vi "XYZStage-move command constructor.vi"(6 "Bypass Z-safety interlock":bool, 9 "Z":sgl, 10 "Y":sgl, 11 "X":sgl) -> (0 "Move command":string, 1 "Adjusted Z":sgl, 2 "Adjusted Y":sgl, 3 "Adjusted X":sgl)   [LabVIEW 2013]
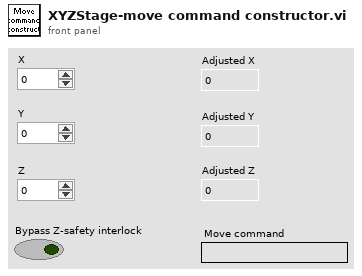
[diagram p1: front panel]
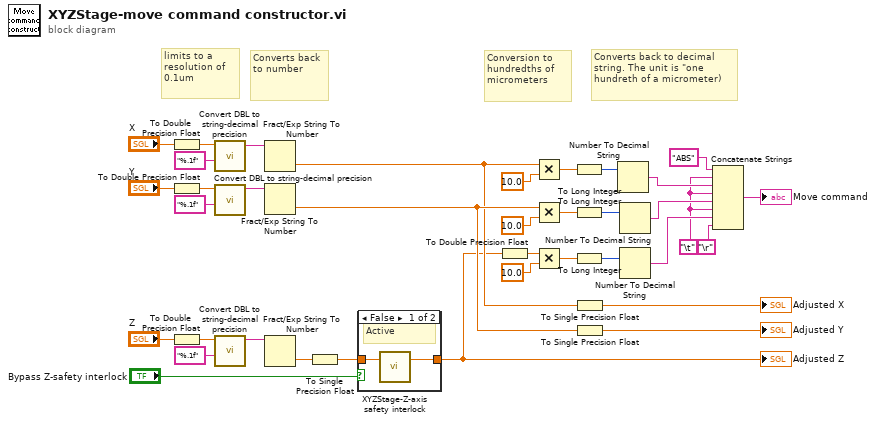
[diagram p0: block diagram]
diagram:
  w17 = "\t" ("Tab Constant")
  # "Converts back to decimal string. The unit is \"one hundreth of a micrometer)"
  # "Converts back to number"
  # "limits to a resolution of 0.1um"
  # "Conversion to hundredths of micrometers"
  n1 = To Double Precision Float(number="X") -> (double precision float=w4:dbl)
  n2 = To Double Precision Float(number="Y") -> (double precision float=w3:dbl)
  n3 = To Double Precision Float(number="Z") -> (double precision float=w2:dbl)
  n4 = call "Convert DBL to string-decimal precision.vi"("Format (%f)"="%.1f", "DBL Value"=w4) -> ("Converted to String"=w28:string)  [unwired: 9 in]
  n5 = call "Convert DBL to string-decimal precision.vi"("Format (%f)"="%.1f", "DBL Value"=w3) -> ("Converted to String"=w29:string)  [unwired: 9 in]
  n6 = call "Convert DBL to string-decimal precision.vi"("Format (%f)"="%.1f", "DBL Value"=w2) -> ("Converted to String"=w30:string)  [unwired: 9 in]
  n7 = Fract/Exp String To Number(string=w28) -> (number=w36:dbl)  [unwired: 3 in, 1 out]
  n8 = Fract/Exp String To Number(string=w29) -> (number=w37:dbl)  [unwired: 3 in, 1 out]
  n9 = Fract/Exp String To Number(string=w30) -> (number=w8:dbl)  [unwired: 3 in, 1 out]
  n10 = To Single Precision Float(number=w8) -> (single precision float=w6:sgl)
  n11 = case shown="False" "Bypass Z-safety interlock" {
    tunnel: [w39 w40] -> w7
    tunnel: w6 -> [w38 w40]
    frame False {
      # "Active"
      n12 = call "XYZStage-Z-axis safety interlock.vi"("Z"=w38) -> ("Z"=w39:sgl)  [unwired: 2 in]
    }
    frame True {
      # "Bypassed"
    }
  }
  "Adjusted Z" <- w7
  n13 = To Double Precision Float(number=w7) -> (double precision float=w5:dbl)
  n14 = Multiply(x=w36, y=10.0) -> (x*y=w12:dbl)
  n15 = Multiply(x=w37, y=10.0) -> (x*y=w32:dbl)
  n16 = Multiply(x=w5, y=10.0) -> (x*y=w34:dbl)
  n17 = To Long Integer(number=w12) -> (32bit integer=w11:i32)
  n18 = To Long Integer(number=w32) -> (32bit integer=w10:i32)
  n19 = To Long Integer(number=w34) -> (32bit integer=w9:i32)
  n20 = To Single Precision Float(number=w36) -> (single precision float=→"Adjusted X":sgl)
  n21 = To Single Precision Float(number=w37) -> (single precision float=→"Adjusted Y":sgl)
  n22 = Number To Decimal String(number=w11) -> (decimal integer string=w31:string)  [unwired: 1 in]
  n23 = Number To Decimal String(number=w10) -> (decimal integer string=w33:string)  [unwired: 1 in]
  n24 = Number To Decimal String(number=w9) -> (decimal integer string=w35:string)  [unwired: 1 in]
  n25 = Concatenate Strings("ABS" ("decimal integer string"), w17, w31, w17, w33, w17, w35, "\r" ("Carriage Return Constant")) -> (→"Move command":string)
